vi "control.vi"() -> ()   [LabVIEW 2009]
uses:
  <vilib>/Instr/_visa.llb/VISA Configure Serial Port (Instr).vi
panel:
  in  "stop":bool
  in  "Frequency (Hz)":dbl
  out "Device":string
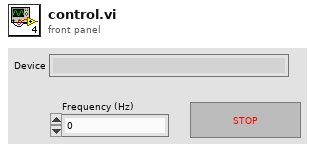
[diagram p1: front panel]
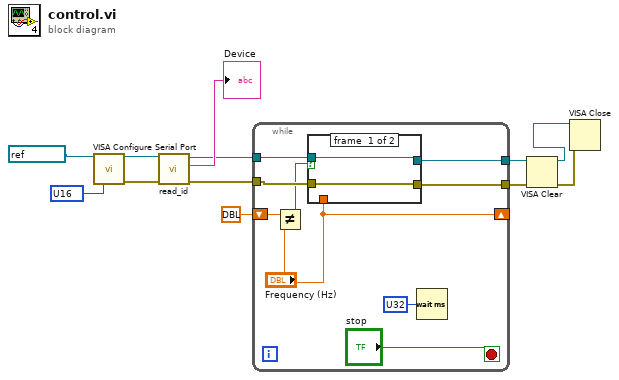
[diagram p0: block diagram]
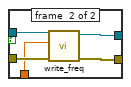
[diagram p2: hidden frame]
diagram:
  w11 = u16 ? items=["1.0", "1.5", "2.0"] ("stop bits (10: 1 bit)")
  n1 = call-poly "VISA Configure Serial Port"("VISA resource name"=refnum<visa-resource-name> ?, "stop bits (10: 1 bit)"=w11) -> ("VISA resource name out"=w10:refnum<visa-resource-name>, "error out"=w9:errorcluster)  [unwired: 12 in]
  n2 = call "read_id.vi"("error in (no error)"=w9, "VISA resource name in"=w10) -> ("error out"=w6:errorcluster, "ID string"=→"Device":string, "VISA resource name out"=w7:refnum<visa-resource-name>)  [unwired: 7 in]
  n3 = while {
    tunnel: w7 -> [w21]
    tunnel: w6 -> [w20]
    tunnel: [w19] -> w5
    tunnel: [w18] -> w3
    shift-right: ["Frequency (Hz)"] -> _
    shift-left: dbl ? ("Frequency (Hz)") -> [w15]
    stop <- "stop" stop-if-true
    n4 = Not Equal?(x=w15, y="Frequency (Hz)") -> (x != y?=w14:bool)
    n5 = case shown="True" w14 {
      tunnel: w21 -> [w23 w28]
      tunnel: w20 -> [w22 w27]
      tunnel: [w22 w26] -> w19
      tunnel: [w23 w25] -> w18
      tunnel: "Frequency (Hz)" -> [_ w24]
      frame #0 {
      }
      frame #1 {
        n6 = call "write_freq.vi"("error in (no error)"=w27, "number"=w24, "VISA Refnum in"=w28) -> ("error out"=w26:errorcluster, "VISA Refnum out"=w25:refnum<visa-resource-name>)  [unwired: 7 in]
      }
    }
    n7 = Wait (ms)(milliseconds to wait=u32 ?) -> ()  [unwired: 1 out]
  }
  n8 = VISA Clear(VISA resource name=w3, error in (no error)=w5) -> (VISA resource name out=w2:refnum<visa-resource-name>, error out=w1:errorcluster)
  n9 = VISA Close(VISA resource name=w2, error in (no error)=w1) -> ()  [unwired: 1 out]
